vi "Write System State.vi"(8 "error in (no error)":errorcluster, 10 "System Status":T1 {"Command Processor Status"."Commands Behind" scale=0.0..10.0; "Command Processor Status"."Queued Commands" scale=0.0..100.0}, 11 "System Actor in":refnum<class "System Actor.lvclass">) -> (0 "error out":errorcluster, 3 "System Actor out":refnum<class "System Actor.lvclass">)   [LabVIEW 2014, in "Robot Actor Framework.lvlib" / "System Actor.lvlib" / "System Actor.lvclass"]
uses:
  System Actor.lvclass
  System State.ctl
  Command Actor/Command Actor Class/Command State.ctl
  Command Actor/Command Actor Class/Command States.ctl
  Command Processor Actor/Command Processor Actor Class/Command Processor State.ctl
  Command Processor Actor/Command Processor Actor Class/Command Processor States.ctl
  System Actor.lvclass/System Actor.ctl
  Command Actor/Command Actor Class/Command Actor.lvclass
  Command Processor Actor/Command Processor Actor Class/Command Processor Actor.lvclass
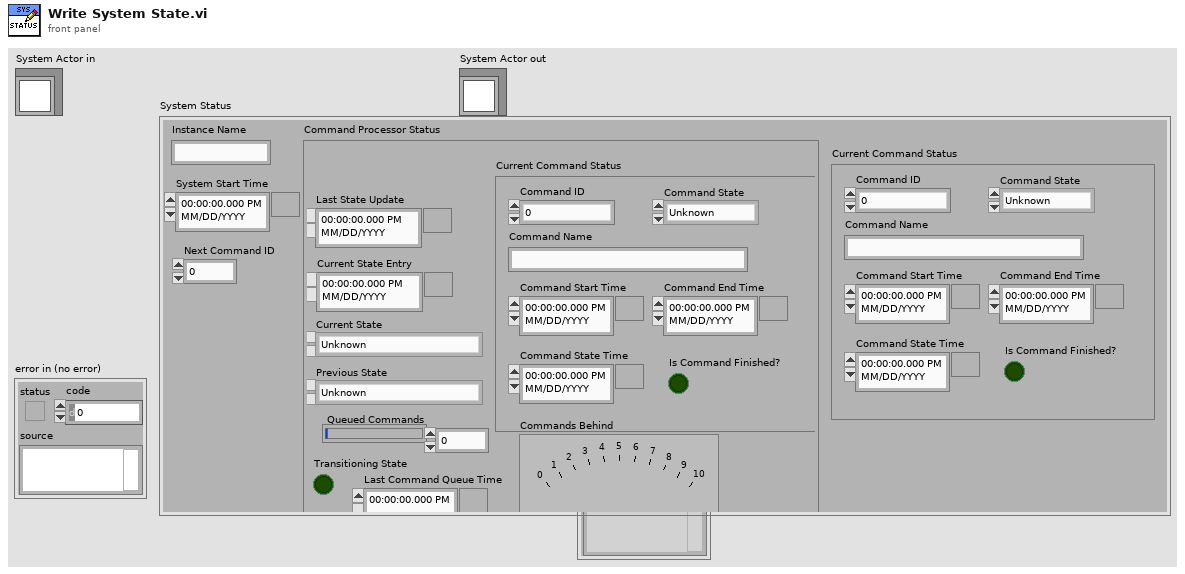
[diagram p1: front panel]
types:
  T1 = typedef "Robot Actor Framework.lvlib/System Actor.lvlib/System Actor.lvclass/System State.ctl" = cluster{"Instance Name":string, "Current Command Status":T2, "System Start Time":timestamp, "Next Command ID":dbl, "Command Processor Status":T4}
  T2 = typedef "Robot Actor Framework.lvlib/Command Actor.lvlib/Command Actor.lvclass/Command State.ctl" = cluster{"Command Name":string, "Command Start Time":timestamp, "Command End Time":timestamp, "Is Command Finished?":bool, "Command ID":u32, "Command State":T3, "Command State Time":timestamp}
  T3 = typedef "Robot Actor Framework.lvlib/Command Actor.lvlib/Command Actor.lvclass/Command States.ctl" = enum16{"Unknown", "Started", "Stopped", "Finished"}
  T4 = typedef "Robot Actor Framework.lvlib/Command Processor Actor.lvlib/Command Processor Actor.lvclass/Command Processor State.ctl" = cluster{"Current State":T5, "Last State Update":timestamp, "Queued Commands":u32, "Current Command Status":T2, "Previous State":T5, "Current State Entry":timestamp, "Transitioning State":bool, "Commands Behind":dbl, "Last Command Queue Time":timestamp}
  T5 = typedef "Robot Actor Framework.lvlib/Command Processor Actor.lvlib/Command Processor Actor.lvclass/Command Processor States.ctl" = enum16{"Unknown", "No Command", "Running Command", "Starting Command", "Stopping Command", "Finishing Command"}
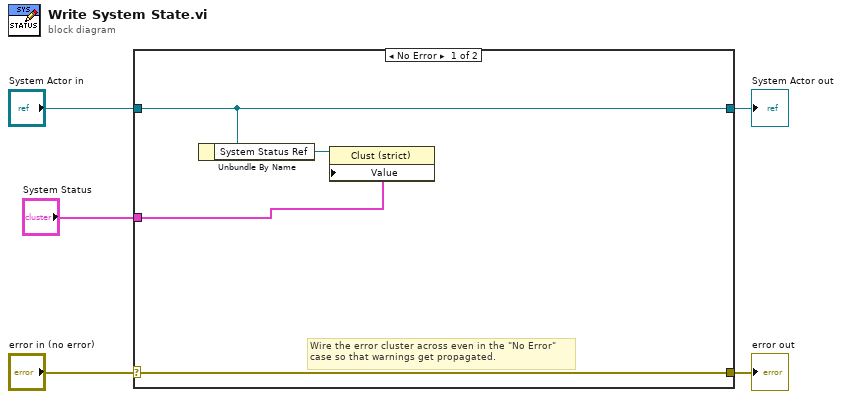
[diagram p0: block diagram]
diagram:
  n1 = case shown="No Error" "error in (no error)" {
    selector: "error in (no error)" -> [w9 w11]
    tunnel: [w9 w11] -> w4
    tunnel: [w8 w10] -> w2
    tunnel: "System Actor in" -> [w8 w10]
    tunnel: "System Status" -> [w6 _]
    frame No Error {
      # "Wire the error cluster across even in the \"No Error\"\ncase so that warnings get propagated."
      n2 = Unbundle By Name(w8) -> ("System Status Ref"=w7:refnum<vi>)
      n3 = property class="Clust (strict)"(reference=w7, "Value"=w6) -> ()  [unwired: 1 in, 2 out]
    }
    frame Error {
    }
  }
  "error out" <- w4
  "System Actor out" <- w2
